vi "LCP Get Valve Handle.vi"(8 "error in (no error)":errorcluster caption="Fehler (Eingang, kein Fehler)", 11 "Pump Handle":i64) -> (0 "error out":errorcluster caption="Fehler (Ausgang)", 3 "Valve Handle":i64)   [LabVIEW 2021, in "labbCAN_Pump_API.lvlib"]
doc: "LCP_Func long LCP_CALL LCP_GetValveHandle(dev_hdl hPump);"
uses:
  labbCAN_Pump_API.lvlib
  labbCAN_Pump_API.dll
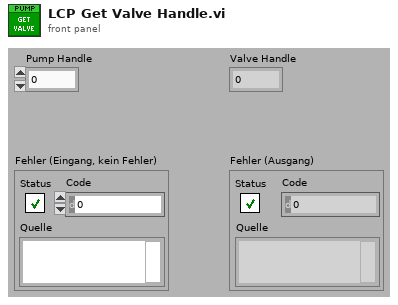
[diagram p1: front panel]
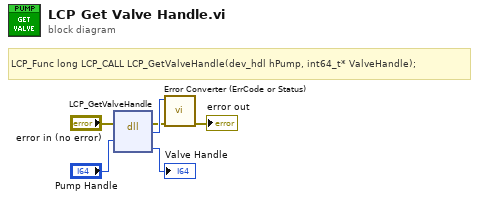
[diagram p0: block diagram]
diagram:
  # "LCP_Func long LCP_CALL LCP_GetValveHandle(dev_hdl hPump, int64_t* ValveHandle);"
  n1 = dll-call lib="C:/Users/olaja/AppData/Local/CETONI_SDK/labbCAN_Pump_API.*" fn="LCP_GetValveHandle"(error in="error in (no error)", "hPump"="Pump Handle") -> (error out=w3:errorcluster, "Rückgabetyp"=w6:i32, "ValveHandle"=→"Valve Handle":i64)  [unwired: 4 in, 1 out]
  n2 = call "Error Converter (ErrCode or Status).vi"("error in (no error)"=w3, "error code"=w6) -> ("error out"=→"error out":errorcluster)  [unwired: 9 in]
